vi "Main.vi"(8 "error in (no error)":errorcluster, 11 "focusBase in":refnum<class "focus.lvclass">) -> (0 "error out":errorcluster, 3 "component":refnum<class "focus.lvclass">)   [LabVIEW 2012, in "focus.lvclass"]
doc: "Main VI of the component."
uses:
  focus.lvclass
  <vilib>/Distrio/Murmex/Murmex/command_enum.ctl
  focus.lvclass/focus.ctl
  <vilib>/Distrio/Murmex/InitialiseMessage/InitialiseMessage.lvclass
  <vilib>/Distrio/Murmex/GenericMessage/GenericMessage.lvclass
  <vilib>/Distrio/Murmex/StopMessage/StopMessage.lvclass
  <vilib>/Distrio/Murmex/ConfigureMessage/ConfigureMessage.lvclass
  <vilib>/Distrio/Murmex/TerminateMessage/TerminateMessage.lvclass
  <vilib>/Distrio/Murmex/Murmex/update_cluster.ctl
  <vilib>/Distrio/Murmex/Murmex/Set configure at initialise.vi
  <vilib>/Distrio/Murmex/Murmex/Set log reference.vi
  <vilib>/Distrio/Murmex/Murmex/Set VI reference.vi
  <vilib>/Distrio/Murmex/Murmex/Get ID.vi
  <vilib>/Distrio/Murmex/Murmex/Murmex.lvclass
  <vilib>/Distrio/Murmex/Message/Message.lvclass
panel:
  out "terminate?":bool=TRUE
  in  "Tab Control":enum32{"Main", "Debug"}(tab)
  out "current Zeta":dbl[unit]
  in  "speedZeta":dbl[unit]
  in  "forwardzeta":bool
  in  "stepzeta":dbl[unit]
  in  "backzeta":bool
  in  "targetZeta":dbl[unit]
  in  "Generic command":string
  in  "command":T1
  in  "button::send":bool
  out "log":string
  in  "button::configure":bool
  in  "button::stop":bool
  in  "button::quit":bool
  in  "ID":string="stage"
  # "Current\nposition"
  # "Target\nposition"
  # "Speed"
  # "Steps"
  # "Zeta"
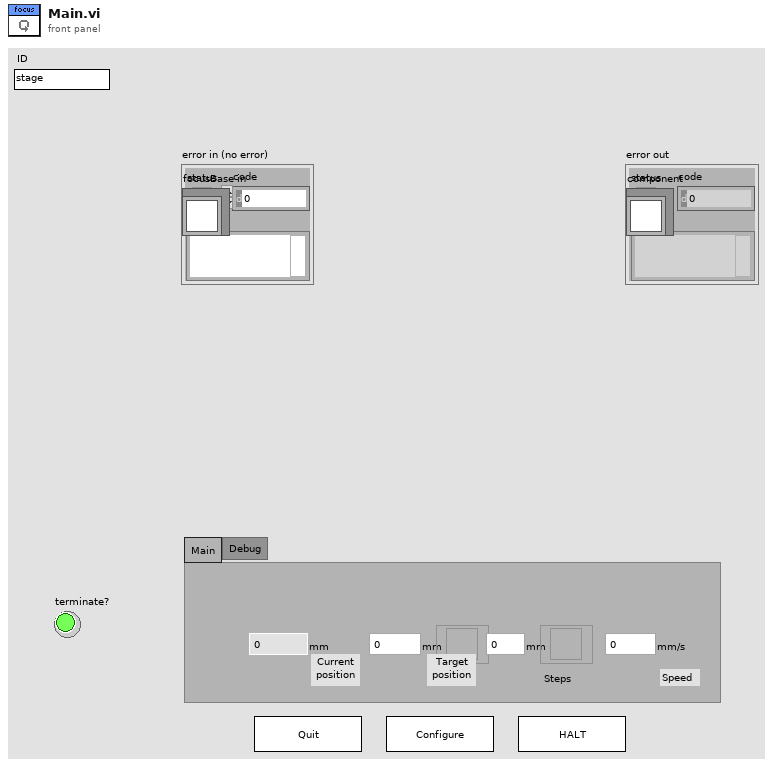
[diagram p1: front panel]
types:
  T1 = typedef "Murmex.lvlib/Murmex.lvclass/command_enum.ctl" = enum16{"null", "initialise", "reset", "terminate", "acknowledge", "update", "inspect", "inform", "proceed", "start", "stop", "fetch", "configure", "generic"}
  T2 = enum8{"Enabled", "Disabled", "Disabled and Grayed Out"}
  T3 = typedef "Murmex.lvlib/Murmex.lvclass/update_cluster.ctl" = cluster{"target ID":string, "key chains":string[], "values":variant[]}
  T4 = typedef "Murmex.lvlib/Murmex.lvclass/Event type enumerations.ctl" = enum16{"before", "after"}
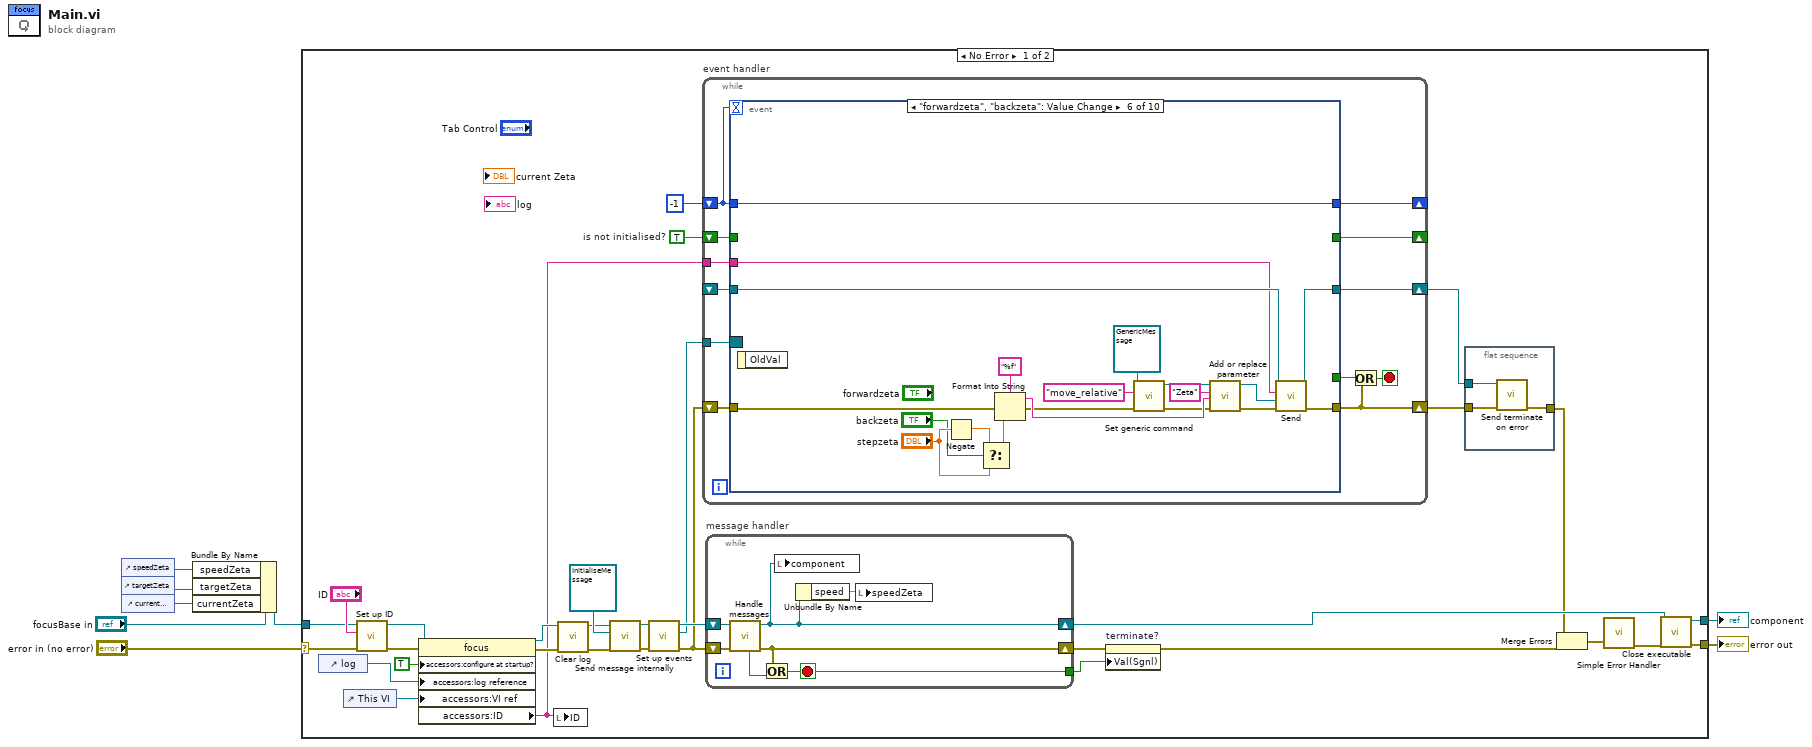
[diagram p0: block diagram]
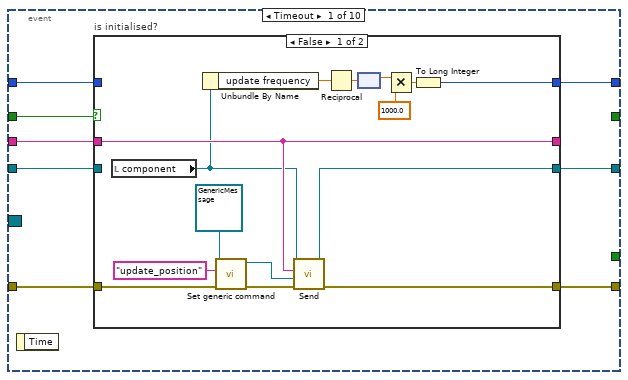
[diagram p2: hidden frame]
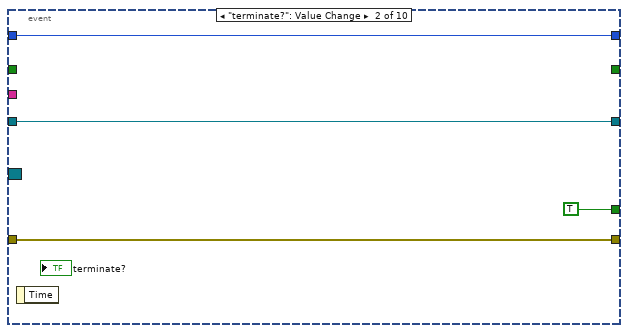
[diagram p4: hidden frame]
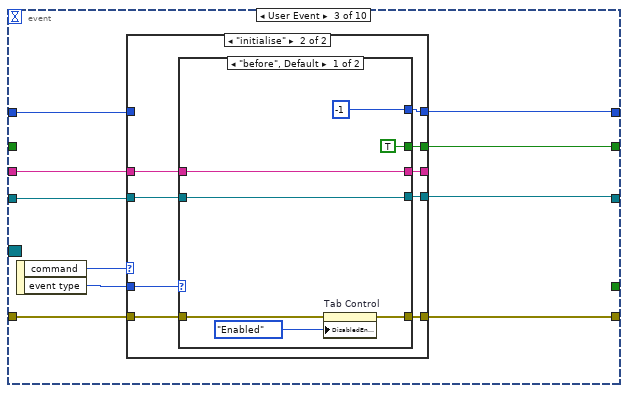
[diagram p5: hidden frame]
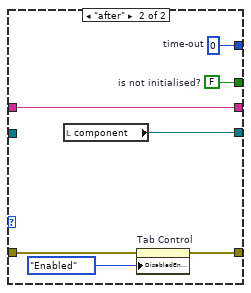
[diagram p7: hidden frame]
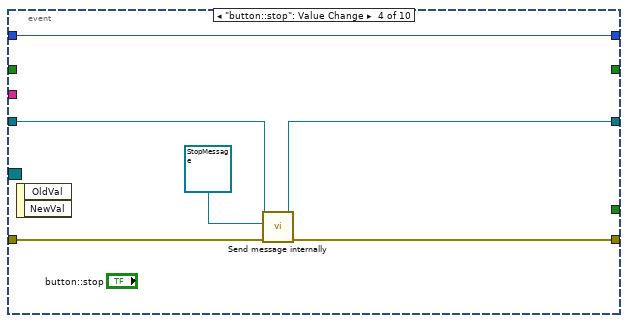
[diagram p8: hidden frame]
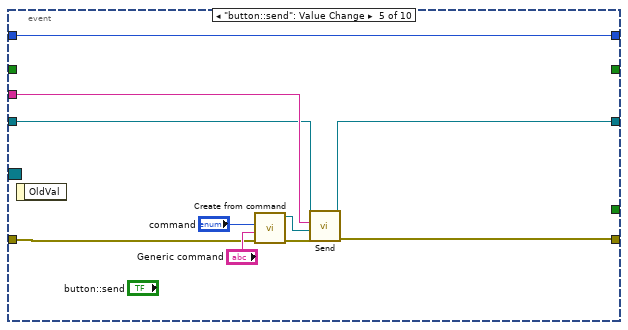
[diagram p9: hidden frame]
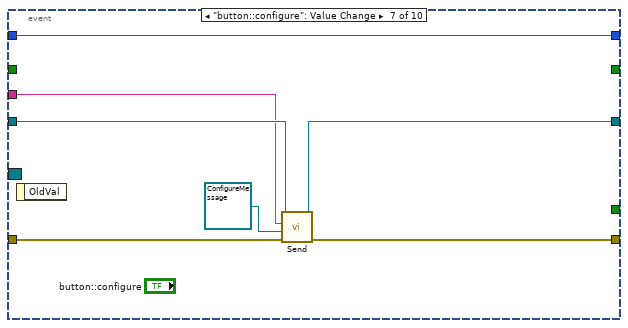
[diagram p10: hidden frame]
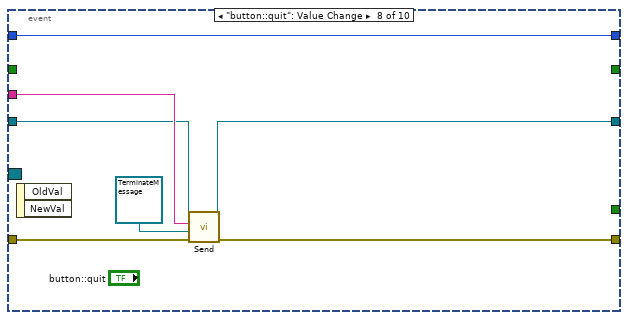
[diagram p11: hidden frame]
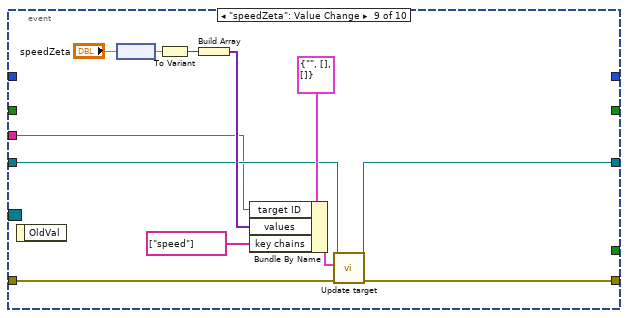
[diagram p12: hidden frame]
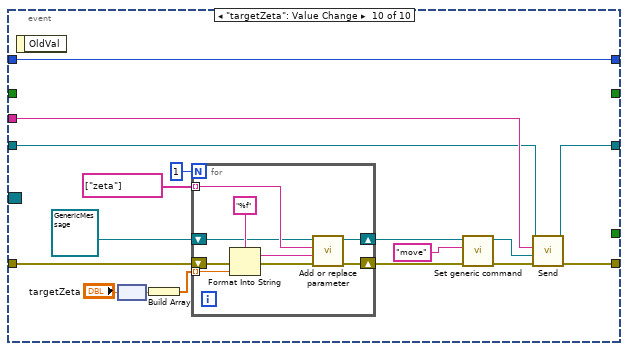
[diagram p13: hidden frame]
diagram:
  n1 = control-ref of="speedZeta"() -> (w1:refnum<vi>)
  n2 = control-ref of="targetZeta"() -> (w2:refnum<vi>)
  n3 = control-ref of="current Zeta"() -> (w3:refnum<vi>)
  n4 = Bundle By Name(cluster="focusBase in", "speedZeta"=w1, "targetZeta"=w2, "currentZeta"=w3) -> (w6:refnum<class "focus.lvclass">)
  n5 = case shown="No Error" "error in (no error)" {
    selector: "error in (no error)" -> [w39 w220]
    tunnel: w6 -> [w38 w219]
    tunnel: [w18 w220] -> w5
    tunnel: [w17 w219] -> w4
    frame No Error {
      w14 = TRUE  # is not initialised?
      n6 = control-ref of="log"() -> (w9:refnum<vi>)
      n7 = control-ref of="This VI"() -> (w34:refnum<vi>)
      n8 = call <vilib>:"Set up ID.vi"("error in (no error)"=w39, "component ID"="ID", "MurmexBase in"=w38) -> ("error out"=w37:errorcluster, "MurmexBase out"=w36:refnum<class "focus.lvclass">)  [unwired: 6 in, 1 out]
      n9 = property class="focus"(reference=w36, error in=w37, "accessors:configure at startup?"=TRUE ("configure at startup?"), "accessors:log reference"=w9, "accessors:VI ref"=w34) -> (reference out=w27:refnum<class "focus.lvclass">, error out=w28:errorcluster, "accessors:ID"=w12:string)
      n10 = local write "ID"(w12) -> ()
      n11 = call <vilib>:"Clear log.vi"("error in (no error)"=w28, "MurmexBase in"=w27) -> ("error out"=w29:errorcluster, "MurmexBase out"=w30:refnum<class "focus.lvclass">)  [unwired: 8 in]
      n12 = call <vilib>:"Send message internally.vi"("error in (no error)"=w29, "Message"=refnum<class "InitialiseMessage.lvclass"> refnum ("Distrio Murmex 1.1:InitialiseMessage"), "Murmex in"=w30) -> ("error out"=w32:errorcluster, "Murmex out"=w33:refnum<class "focus.lvclass">)  [unwired: 7 in]
      n13 = call <vilib>:"Set up events.vi"("error in (no error)"=w32, "MurmexBase in"=w33) -> ("error out"=w16:errorcluster, "Event Registration Refnum"=w15:refnum<event-registration>, "MurmexBase out"=w26:refnum<class "focus.lvclass">)  [unwired: 7 in]
      n14 = while "event handler" {
        shift-right: [w44] -> w10
        shift-left: w16 -> [w52]
        tunnel: w15 -> [w51]
        shift-right: [w41] -> _
        shift-left: w14 -> [w50]
        shift-right: [w45] -> _
        shift-left: -1 -> [w49]
        tunnel: w12 -> [w48]
        shift-right: [w47] -> w11
        shift-left: _ -> [w46]
        stop <- w42 stop-if-true
        n15 = event shown="[5] \"forwardzeta\", \"backzeta\": Value Change" {
          selector: w51 -> [_ _ _ _ _ _ _ _ _ _]
          dyn-events: _ -> [_ _ _ _ _ _ _ _ _ _]
          timeout: w49 -> [_ _ _ _ _ _ _ _ _ _]
          tunnel: w52 -> [w59 w80 w93 w125 w132 w143 w162 w169 w178 w196]
          tunnel: w50 -> [w53 _ _ _ _ _ _ _ _ _]
          tunnel: w49 -> [w60 w83 w88 w123 w127 w137 w157 w164 _ w187]
          tunnel: w48 -> [w58 _ w87 _ w130 w138 w158 w167 w171 w186]
          tunnel: [w57 w80 w84 w124 w131 w144 w161 w168 w177 w189] -> w44
          tunnel: [w56 w82 w91 w121 w128 w139 w159 w165 w174 w184] -> w47
          tunnel: w46 -> [w55 w82 w92 w122 w129 w140 w160 w166 w175 w185]
          tunnel: [w54 w83 w86 w123 w127 w137 w157 w164 _ w187] -> w45
          tunnel: [_ TRUE _ _ _ _ _ _ _ _] -> w43
          tunnel: [_ _ w85 _ _ _ _ _ _ _] -> w41
          event Timeout {
            n16 = event-data() -> ()  [unwired: 1 in, 1 out]
            n17 = case "is initialised?" shown="False" w53 {
              tunnel: w60 -> [_ w79]
              tunnel: w59 -> [w71 w76]
              tunnel: w58 -> [w70 w78]
              tunnel: [w70 w78] -> _
              tunnel: [w69 w76] -> w57
              tunnel: [w68 w77] -> w56
              tunnel: w55 -> [_ w77]
              tunnel: [w61 w79] -> w54
              frame False {
                n18 = local read "component"() -> (w67:refnum<class "focus.lvclass">)
                n19 = Unbundle By Name(w67) -> ("update frequency"=w62:dbl[unit])
                n20 = call <vilib>:"Set generic command.vi"("error in (no error)"=w71, "generic command"="update_position", "GenericMessage in"=refnum<class "GenericMessage.lvclass"> refnum ("Distrio Murmex 1.1:GenericMessage")) -> ("error out"=w74:errorcluster, "GenericMessage out"=w75:refnum<class "GenericMessage.lvclass">)  [unwired: 7 in]
                n21 = call <vilib>:"Send.vi"("error in (no error)"=w74, "Message"=w75, "recipient"=w70, "Murmex in"=w67) -> ("error out"=w69:errorcluster, "Murmex out"=w68:refnum<class "focus.lvclass">)  [unwired: 6 in]
                n22 = Reciprocal(x=w62) -> (1/x=w63:dbl[unit])
                n23 = node(w63) -> (w65:dbl)
                n24 = Multiply(x=w65, y=1000.0) -> (x*y=w66:dbl)
                n25 = To Long Integer(number=w66) -> (32bit integer=w61:i32)
              }
              frame True {
              }
            }
          }
          event "terminate?": Value Change {
            n26 = event-data() -> ()  [unwired: 1 in, 1 out]
          }
          event User Event {
            n27 = event-data() -> ("command"=w90:T1, "event type"=w89:T4)  [unwired: 1 in]
            n28 = case shown="\"initialise\"" w90 {
              tunnel: w93 -> [w95 w106]
              tunnel: [w95 w105] -> w84
              tunnel: w87 -> [w97 w104]
              tunnel: [w96 w103] -> w91
              tunnel: w92 -> [w96 w102]
              tunnel: [w97 w101] -> _
              tunnel: w89 -> [_ w100]
              tunnel: [w94 w99] -> w86
              tunnel: w88 -> [w94 _]
              tunnel: [_ w98] -> w85
              frame "null", Default {
              }
              frame "initialise" {
                n29 = case shown="\"before\", Default" w100 {
                  tunnel: [w112 w119] -> w105
                  tunnel: w106 -> [w113 w120]
                  tunnel: w104 -> [w110 w116]
                  tunnel: [w109 w118] -> w103
                  tunnel: w102 -> [w109 _]
                  tunnel: [w110 w116] -> w101
                  tunnel: [-1 w115] -> w99
                  tunnel: [TRUE ("is not initialised?") w114] -> w98
                  frame "before", Default {
                    n30 = property on="Tab Control" class="TabCtl (strict)"(error in=w113, "DisabledEnum"=T2."Enabled" ("Disabled")) -> (error out=w112:errorcluster)  [unwired: 1 in, 1 out]
                  }
                  frame "after" {
                    w114 = FALSE  # is not initialised?
                    w115 = 0  # time-out
                    n31 = local read "component"() -> (w118:refnum<class "focus.lvclass">)
                    n32 = property on="Tab Control" class="TabCtl (strict)"(error in=w120, "DisabledEnum"=T2."Enabled" ("Disabled")) -> (error out=w119:errorcluster)  [unwired: 1 in, 1 out]
                  }
                }
              }
            }
          }
          event "button::stop": Value Change {
            n33 = event-data() -> ()  [unwired: 1 in, 2 out]
            n34 = call <vilib>:"Send message internally.vi"("error in (no error)"=w125, "Message"=refnum<class "StopMessage.lvclass"> refnum ("Distrio Murmex 1.5:StopMessage"), "Murmex in"=w122) -> ("error out"=w124:errorcluster, "Murmex out"=w121:refnum<class "focus.lvclass">)  [unwired: 7 in]
          }
          event "button::send": Value Change {
            n35 = event-data() -> ()  [unwired: 1 in, 1 out]
            n36 = call <vilib>:"Create from command.vi"("error in (no error)"=w132, "generic command"="Generic command", "command"="command") -> ("error out"=w135:errorcluster, "Message out"=w134:refnum<class "Message.lvclass">)  [unwired: 7 in]
            n37 = call <vilib>:"Send.vi"("error in (no error)"=w135, "Message"=w134, "recipient"=w130, "Murmex in"=w129) -> ("error out"=w131:errorcluster, "Murmex out"=w128:refnum<class "focus.lvclass">)  [unwired: 6 in]
          }
          event "forwardzeta", "backzeta": Value Change {
            n38 = event-data() -> ()  [unwired: 1 in, 1 out]
            n39 = Negate(x="stepzeta") -> (-x=w150:dbl[unit])
            n40 = Select(t=w150, s="backzeta", f="stepzeta") -> (s? t:f=w155:dbl[unit])
            n41 = Format Into String(format string="%f", error in=w143, w155) -> (resulting string=w154:string, error out=w151:errorcluster)  [unwired: 1 in]
            n42 = call <vilib>:"Set generic command.vi"("error in (no error)"=w151, "generic command"="move_relative", "GenericMessage in"=refnum<class "GenericMessage.lvclass"> refnum ("Distrio Murmex 1.1:GenericMessage")) -> ("error out"=w146:errorcluster, "GenericMessage out"=w148:refnum<class "GenericMessage.lvclass">)  [unwired: 7 in]
            n43 = call <vilib>:"Add or replace parameter.vi"("error in (no error)"=w146, "value"=w154, "name"="Zeta", "Message in"=w148) -> ("error out"=w147:errorcluster, "Message out"=w153:refnum<class "GenericMessage.lvclass">)  [unwired: 6 in]
            n44 = call <vilib>:"Send.vi"("error in (no error)"=w147, "Message"=w153, "recipient"=w138, "Murmex in"=w140) -> ("error out"=w144:errorcluster, "Murmex out"=w139:refnum<class "focus.lvclass">)  [unwired: 6 in]
          }
          event "button::configure": Value Change {
            n45 = event-data() -> ()  [unwired: 1 in, 1 out]
            n46 = call <vilib>:"Send.vi"("error in (no error)"=w162, "Message"=refnum<class "ConfigureMessage.lvclass"> refnum ("Distrio Murmex 1.1:ConfigureMessage"), "recipient"=w158, "Murmex in"=w160) -> ("error out"=w161:errorcluster, "Murmex out"=w159:refnum<class "focus.lvclass">)  [unwired: 6 in]
          }
          event "button::quit": Value Change {
            n47 = event-data() -> ()  [unwired: 1 in, 2 out]
            n48 = call <vilib>:"Send.vi"("error in (no error)"=w169, "Message"=refnum<class "TerminateMessage.lvclass"> refnum ("Murmex.lvlib:TerminateMessage"), "recipient"=w167, "Murmex in"=w166) -> ("error out"=w168:errorcluster, "Murmex out"=w165:refnum<class "focus.lvclass">)  [unwired: 6 in]
          }
          event "speedZeta": Value Change {
            n49 = event-data() -> ()  [unwired: 1 in, 1 out]
            n50 = node("speedZeta") -> (w182:dbl)
            n51 = To Variant(anything=w182) -> (Variant=w181:variant)
            n52 = Build Array(w181) -> (w176:variant[])
            n53 = Bundle By Name(cluster=T3 {"target ID"="", "key chains"=[], "values"=[]} ("update cluster"), "target ID"=w171, "values"=w176, "key chains"=string[] ["speed"]) -> (w179:T3)
            n54 = call <vilib>:"Update target.vi"("error in (no error)"=w178, "update cluster"=w179, "MurmexBase in"=w175) -> ("error out"=w177:errorcluster, "MurmexBase out"=w174:refnum<class "focus.lvclass">)  [unwired: 7 in]
          }
          event "targetZeta": Value Change {
            n55 = event-data() -> ()  [unwired: 1 in, 1 out]
            n56 = node("targetZeta") -> (w198:dbl)
            n57 = Build Array(w198) -> (w194:dbl[])
            n58 = for {
              N: 1 -> [_]
              shift-right: [w206] -> w190
              shift-left: w196 -> [w205]
              tunnel: string[] ["zeta"] -> [w204] mode=indexing
              shift-right: [w202] -> w188
              shift-left: refnum<class "GenericMessage.lvclass"> refnum ("Distrio Murmex 1.1:GenericMessage") -> [w203]
              tunnel: w194 -> [w201] mode=indexing
              n59 = Format Into String(format string="%f", error in=w205, w201) -> (resulting string=w200:string, error out=w207:errorcluster)  [unwired: 1 in]
              n60 = call <vilib>:"Add or replace parameter.vi"("error in (no error)"=w207, "value"=w200, "name"=w204, "Message in"=w203) -> ("error out"=w206:errorcluster, "Message out"=w202:refnum<class "GenericMessage.lvclass">)  [unwired: 6 in]
            }
            n61 = call <vilib>:"Set generic command.vi"("error in (no error)"=w190, "generic command"="move", "GenericMessage in"=w188) -> ("error out"=w191:errorcluster, "GenericMessage out"=w192:refnum<class "GenericMessage.lvclass">)  [unwired: 7 in]
            n62 = call <vilib>:"Send.vi"("error in (no error)"=w191, "Message"=w192, "recipient"=w186, "Murmex in"=w185) -> ("error out"=w189:errorcluster, "Murmex out"=w184:refnum<class "focus.lvclass">)  [unwired: 6 in]
          }
        }
        n63 = Or(x=w43, y=w44) -> (x .or. y?=w42:bool)
      }
      n64 = while "message handler" {
        shift-right: [w215] -> w25
        shift-left: w16 -> [w217]
        shift-right: [w213] -> w20
        shift-left: w26 -> [w216]
        tunnel: [w214] -> w24
        stop <- w214 stop-if-true
        n65 = call <vilib>:"Handle messages.vi"("error in (no error)"=w217, "Murmex in"=w216) -> ("error out"=w215:errorcluster, "Murmex out"=w213:refnum<class "focus.lvclass">, "terminated?"=w218:bool)  [unwired: 7 in]
        n66 = Or(x=w215, y=w218) -> (x .or. y?=w214:bool)
        n67 = local write "component"(w213) -> ()
        n68 = Unbundle By Name(w213) -> ("speed"=w212:dbl[unit])
        n69 = local write "speedZeta"(w212) -> ()
      }
      n70 = property on="terminate?" class="Bool (strict)"(error in=w25, "Val(Sgnl)"=w24) -> (error out=w21:errorcluster)  [unwired: 1 in, 1 out]
      n71 = flat-sequence {
        tunnel: w10 -> [w211]
        tunnel: [w210] -> w19
        tunnel: w11 -> [w209]
        frame #0 {
          n72 = call <vilib>:"Send terminate on error.vi"("error in (no error)"=w211, "Murmex in"=w209) -> ("error out"=w210:errorcluster)  [unwired: 8 in, 1 out]
        }
      }
      n73 = Merge Errors(w19, w21) -> (w22:errorcluster)
      n74 = call <vilib>:"Simple Error Handler.vi"("error in (no error)"=w22) -> ("error out"=w23:errorcluster)  [unwired: 4 in, 4 out]
      n75 = call <vilib>:"Close executable.vi"("error in (no error)"=w23, "MurmexBase in"=w20) -> ("error out"=w18:errorcluster, "MurmexBase out"=w17:refnum<class "focus.lvclass">)  [unwired: 8 in]
    }
    frame Error {
    }
  }
  "error out" <- w5
  "component" <- w4
